vi "Pin Position Facade.vi"(0 "Data In":T6, 2 "Display State In":T3, 3 "Container State":T5) -> (6 "Data Out":T6, 7 "Display State Out":T3, 8 "Action":T2)   [LabVIEW 2013, in "Pin Position.xctl"]
uses:
  Pin Position.xctl
  Popups/Selected Pin Positions.ctl
  Pin Position Data.ctl
  lib/Data Access Objects/Metadata/Pin Positions.ctl
  <vilib>/_xctls/Container State.ctl
  Pin Position State.ctl
  lib/Data Access Objects/Application/Number Of LBCBs.ctl
  <vilib>/_xctls/Action.ctl
  lib/Data Access Objects/Metadata/Persistant DAO Actions.ctl
  lib/Data Access Objects/Metadata/LBCB Number.ctl
  <vilib>/_xctls/XControlSupport.lvlib
panel:
  in  "LBCB Position Tab":enum32{"LBCB 1", "LBCB 2"}(tab)
  in  "LBCB Position L1":T1
  in  "LBCB Position L2":T1
  # "Fixed"
  # "Platten"
  # "X"
  # "Z"
  # "X"
  # "Z"
  # "Y"
  # "Y"
  # "Fixed"
  # "Platten"
  # "X"
  # "Z"
  # "X"
  # "Z"
  # "Y"
  # "Y"
  # "Fixed"
  # "Platten"
  # "X"
  # "Z"
  # "X"
  # "Z"
  # "Y"
  # "Y"
  # "Fixed"
  # "Platten"
  # "X"
  # "Z"
  # "X"
  # "Z"
  # "Y"
  # "Y"
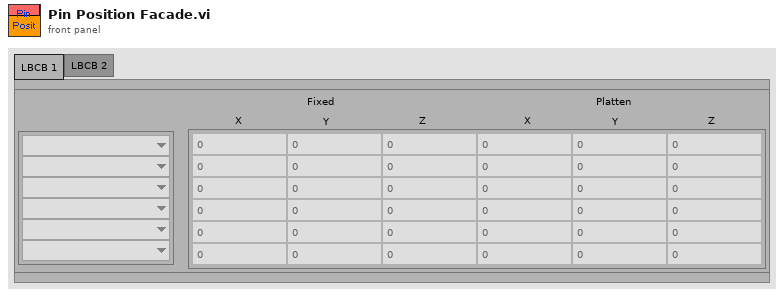
[diagram p1: front panel]
types:
  T1 = typedef "Selected Pin Positions.ctl" = cluster{"Pin Positions":dbl[][], "Row Labels":u16[]}
  T2 = typedef "XControlSupport.lvlib/Action.ctl" = cluster{"Data Changed?":bool, "State Changed?":bool, "Action Name":string}
  T3 = typedef "Pin Position.xctl/Pin Position State.ctl" = cluster{"Number of LBCBs":T4}
  T4 = typedef "Number Of LBCBs.ctl" = enum16{"1", "2"}
  T5 = typedef "XControlSupport.lvlib/Container State.ctl" = cluster{"Indicator?":bool, "Run Mode?":bool, " Refnum":refnum<vi>}
  T6 = typedef "Pin Position.xctl/Pin Position Data.ctl" = T7[]
  T7 = typedef "Pin Positions.ctl" = cluster{"Pin Positions":dbl[][], "Row Labels":string[]}
  T8 = enum8{"Enabled", "Disabled", "Disabled and Grayed Out"}
  T9 = typedef "LBCB Number.ctl" = enum16{"LBCB1", "LBCB2"}
  T10 = typedef "Persistant DAO Actions.ctl" = enum16{"Init", "Get", "Set", "Load", "Save"}
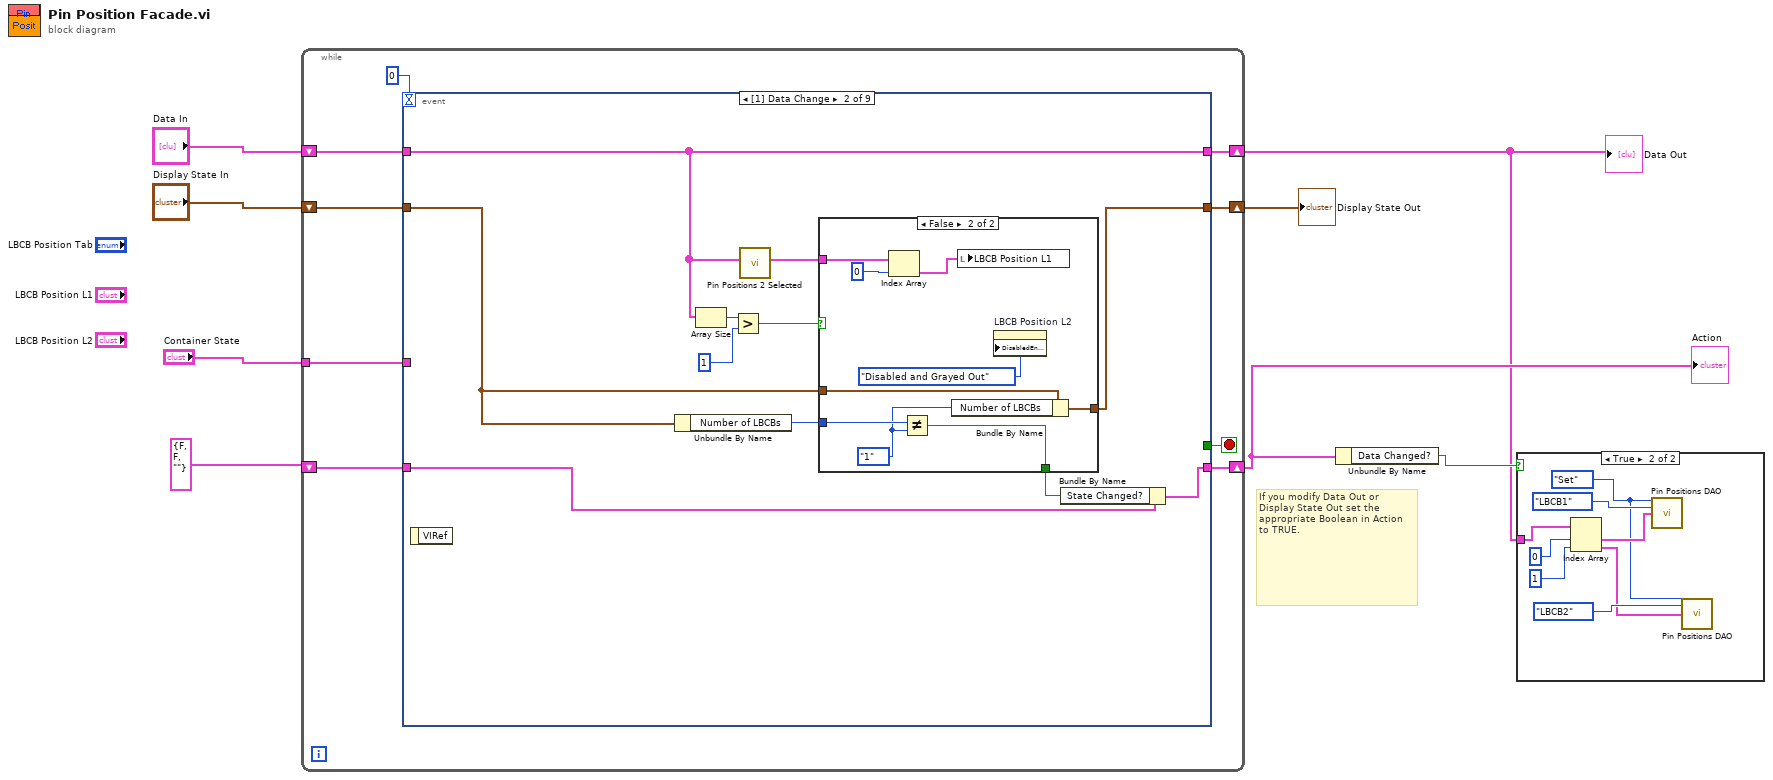
[diagram p0: block diagram]
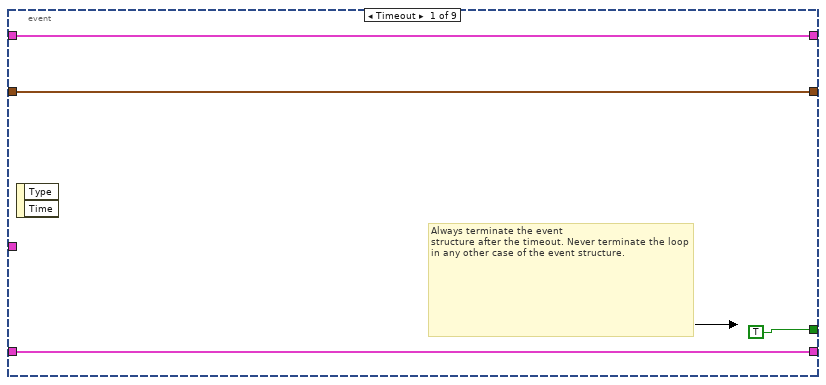
[diagram p3: hidden frame]
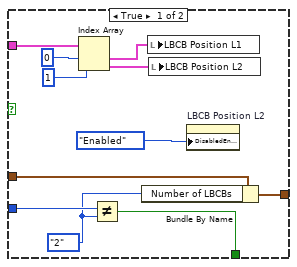
[diagram p4: hidden frame]
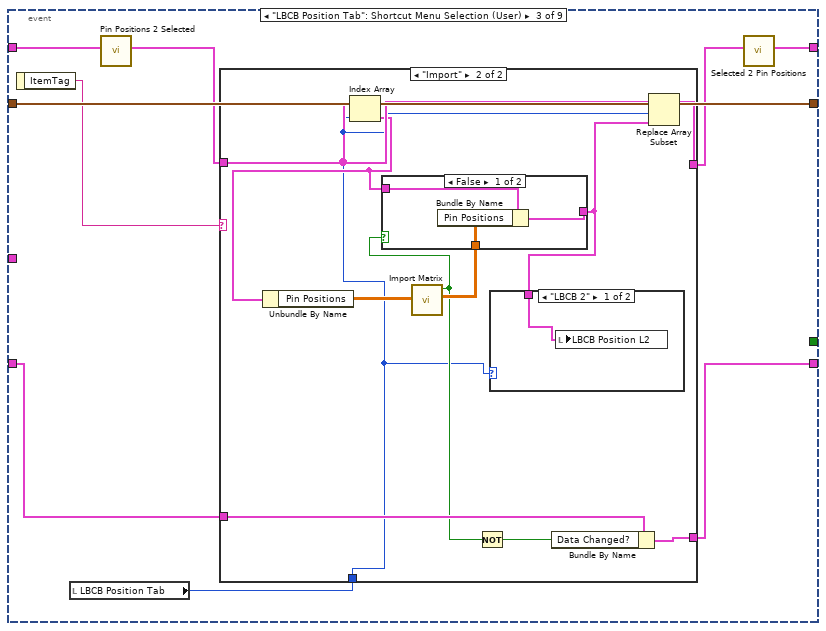
[diagram p5: hidden frame]
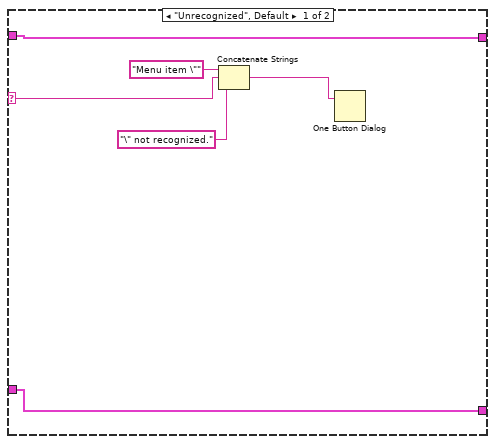
[diagram p6: hidden frame]
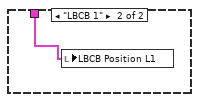
[diagram p7: hidden frame]
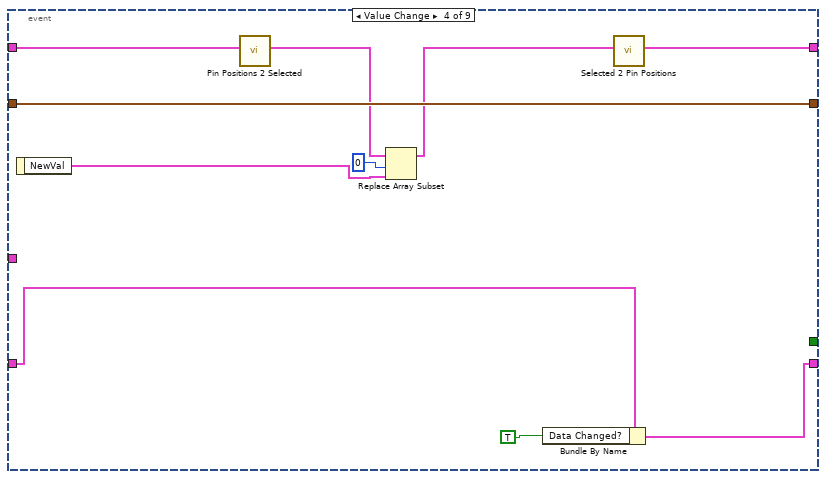
[diagram p9: hidden frame]
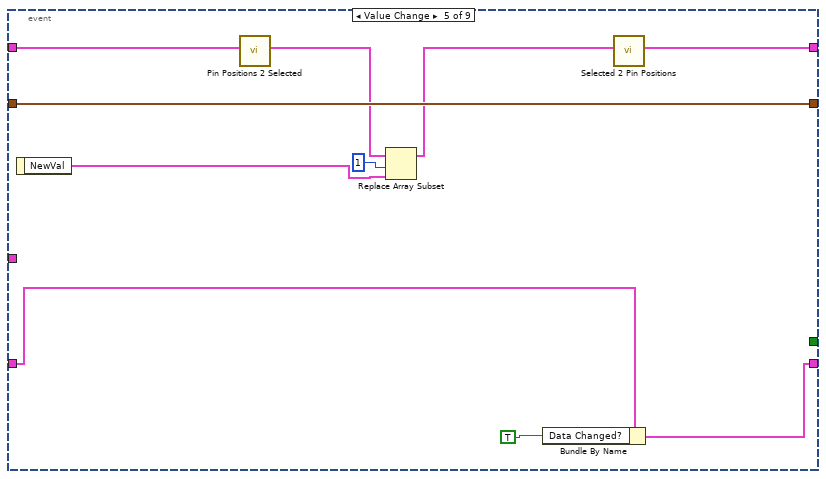
[diagram p10: hidden frame]
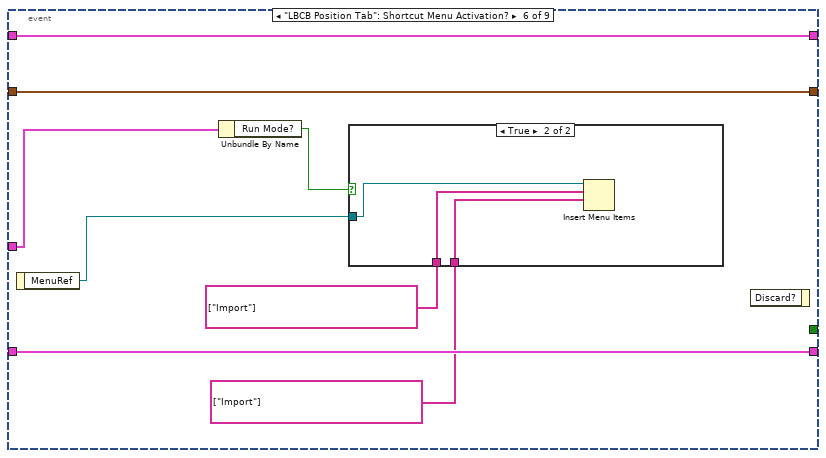
[diagram p11: hidden frame]
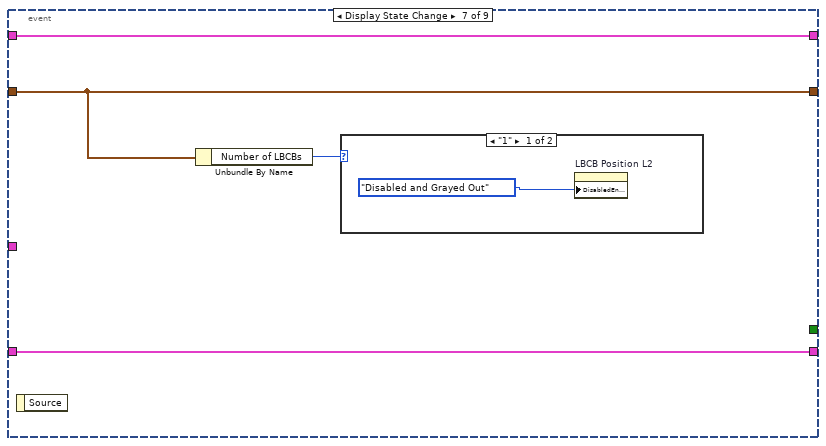
[diagram p13: hidden frame]
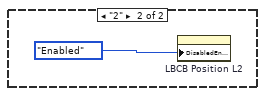
[diagram p14: hidden frame]
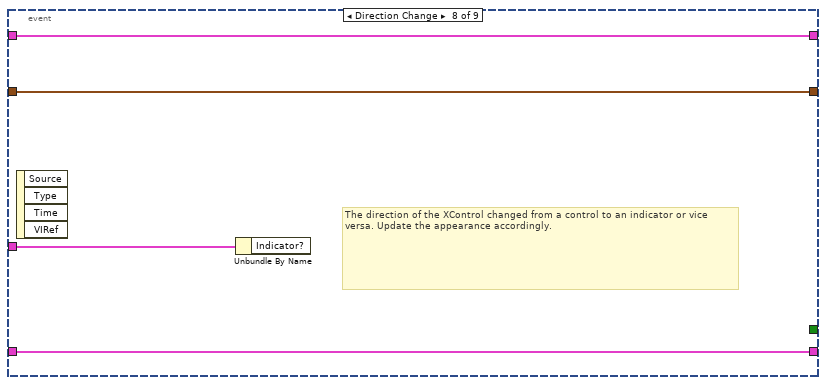
[diagram p15: hidden frame]
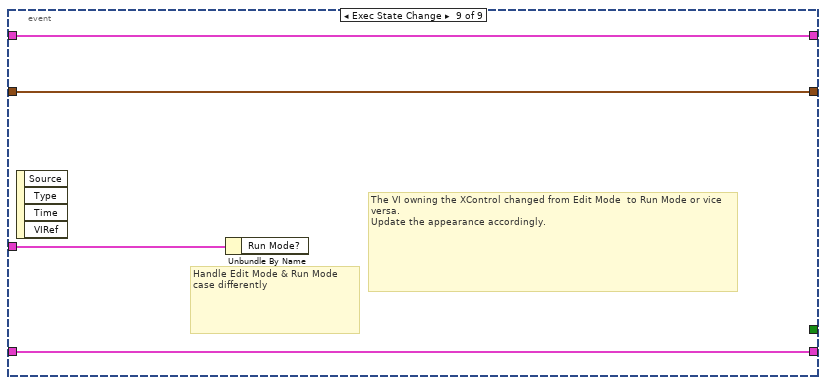
[diagram p16: hidden frame]
diagram:
  # "If you modify Data Out or\nDisplay State Out set the\nappropriate Boolean in Action\nto TRUE."
  n1 = while {
    shift-right: [w16] -> w6
    shift-left: "Display State In" -> [w17]
    tunnel: "Container State" -> [w13]
    shift-right: [w11] -> w1
    shift-left: "Data In" -> [w12]
    shift-right: [w9] -> w2
    shift-left: T2 {"Data Changed?"=FALSE, "State Changed?"=FALSE, "Action Name"=""} ("Action") -> [w10]
    stop <- w15 stop-if-true
    n2 = event shown="[1] Data Change" {
      selector: _ -> [_ _ _ _ _ _ _ _ _]
      dyn-events: _ -> [_ _ _ _ _ _ _ _ _]
      timeout: 0 -> [_ _ _ _ _ _ _ _ _]
      tunnel: w17 -> [w19 w24 w61 w94 w104 w112 w116 w124 w128]
      tunnel: [w19 w23 w61 w94 w104 w112 w116 w124 w128] -> w16
      tunnel: [TRUE _ _ _ _ _ _ _ _] -> w15
      tunnel: w13 -> [_ _ _ _ _ w106 _ w125 w129]
      tunnel: w12 -> [w18 w27 w58 w90 w100 w111 w119 w123 w127]
      tunnel: [w18 w27 w54 w87 w97 w111 w119 w123 w127] -> w11
      tunnel: [w20 w25 w56 w85 w95 w110 w118 w122 w126] -> w9
      tunnel: w10 -> [w20 w26 w60 w86 w96 w110 w118 w122 w126]
      event Timeout {
        # "Always terminate the event\nstructure after the timeout. Never terminate the loop in any other case of the event structure."
        n3 = event-data() -> ()  [unwired: 1 in, 2 out]
      }
      event Data Change {
        n4 = event-data() -> ()  [unwired: 1 in, 1 out]
        n5 = Unbundle By Name(w24) -> ("Number of LBCBs"=w31:T4)
        n6 = Array Size(array=w27) -> (size(s)=w28:i32)
        n7 = Greater?(x=w28, y=1) -> (0:w30:bool)
        n8 = call "Pin Positions 2 Selected.vi"("Pin"=w27) -> ("Selected"=w22:T1[])  [unwired: 10 in]
        n9 = case shown="False" w30 {
          tunnel: w22 -> [w43 w52]
          tunnel: w24 -> [w37 w48]
          tunnel: w31 -> [w38 w49]
          tunnel: [w35 w46] -> w32
          tunnel: [w34 w45] -> w23
          frame True {
            w36 = Number_Of_LBCBs."2" ("y")
            n10 = Index Array(array=w43, index #1=0 ("index"), index #2=1 ("index")) -> (element #1=w40:T1, element #2=w39:T1)
            n11 = Not Equal?(x=w38, y=w36) -> (x != y?=w35:bool)
            n12 = Bundle By Name(cluster=w37, "Number of LBCBs"=w36) -> (w34:T3)
            n13 = local write "LBCB Position L1"(w40) -> ()
            n14 = local write "LBCB Position L2"(w39) -> ()
            n15 = property on="LBCB Position L2" class="Clust (strict)"("DisabledEnum"=T8."Enabled" ("Disabled")) -> ()  [unwired: 2 in, 2 out]
          }
          frame False {
            w47 = Number_Of_LBCBs."1" ("y")
            n16 = Index Array(array=w52, index=0) -> (element=w50:T1)
            n17 = Not Equal?(x=w49, y=w47) -> (x != y?=w46:bool)
            n18 = Bundle By Name(cluster=w48, "Number of LBCBs"=w47) -> (w45:T3)
            n19 = local write "LBCB Position L1"(w50) -> ()
            n20 = property on="LBCB Position L2" class="Clust (strict)"("DisabledEnum"=T8."Disabled and Grayed Out" ("Disabled")) -> ()  [unwired: 2 in, 2 out]
          }
        }
        n21 = Bundle By Name(cluster=w26, "State Changed?"=w32) -> (w25:T2)
      }
      event "LBCB Position Tab": Shortcut Menu Selection (User) {
        n22 = event-data() -> ("ItemTag"=w59:string)  [unwired: 1 in]
        n23 = local read "LBCB Position Tab"() -> (w53:enum32{"LBCB 1", "LBCB 2"})
        n24 = call "Pin Positions 2 Selected.vi"("Pin"=w58) -> ("Selected"=w55:T1[])  [unwired: 10 in]
        n25 = case shown="\"Import\"" w59 {
          selector: w59 -> [w65 _]
          tunnel: w55 -> [w63 w78]
          tunnel: [w63 w77] -> w57
          tunnel: w60 -> [w62 w73]
          tunnel: [w62 w72] -> w56
          tunnel: w53 -> [_ w68]
          frame "Unrecognized", Default {
            n26 = Concatenate Strings("Menu item \"" ("string"), w65, "\" not recognized." ("string")) -> (w64:string)
            n27 = One Button Dialog(message=w64) -> ()  [unwired: 1 in, 1 out]
          }
          frame "Import" {
            n28 = Index Array(array=w78, index=w68) -> (element=w76:T1)
            n29 = Unbundle By Name(w76) -> ("Pin Positions"=w75:dbl[][])
            n30 = call "Import Matrix.vi"("PinPositions In"=w75) -> ("PinPositions Out"=w74:dbl[][], "Canceled"=w71:bool)  [unwired: 9 in]
            n31 = case shown="False" w71 {
              tunnel: [w83 w84] -> w69
              tunnel: w76 -> [w82 w84]
              tunnel: w74 -> [w81 _]
              frame False {
                n32 = Bundle By Name(cluster=w82, "Pin Positions"=w81) -> (w83:T1)
              }
              frame True {
              }
            }
            n33 = Not(x=w71) -> (.not. x?=w70:bool)
            n34 = case shown="\"LBCB 2\"" w68 {
              tunnel: w69 -> [w79 w80]
              frame "LBCB 2" {
                n35 = local write "LBCB Position L2"(w79) -> ()
              }
              frame "LBCB 1" {
                n36 = local write "LBCB Position L1"(w80) -> ()
              }
            }
            n37 = Bundle By Name(cluster=w73, "Data Changed?"=w70) -> (w72:T2)
            n38 = Replace Array Subset(array=w78, new element=w69, index=w68) -> (w77:T1[])
          }
        }
        n39 = call "Selected 2 Pin Positions.vi"("Selected"=w57) -> ("Pin"=w54:T7[])  [unwired: 10 in]
      }
      event Value Change {
        n40 = event-data() -> ("NewVal"=w91:T1)  [unwired: 1 in]
        n41 = call "Pin Positions 2 Selected.vi"("Pin"=w90) -> ("Selected"=w89:T1[])  [unwired: 10 in]
        n42 = Replace Array Subset(array=w89, new element=w91, index=0) -> (w88:T1[])
        n43 = Bundle By Name(cluster=w86, "Data Changed?"=TRUE) -> (w85:T2)
        n44 = call "Selected 2 Pin Positions.vi"("Selected"=w88) -> ("Pin"=w87:T7[])  [unwired: 10 in]
      }
      event Value Change {
        n45 = event-data() -> ("NewVal"=w101:T1)  [unwired: 1 in]
        n46 = call "Pin Positions 2 Selected.vi"("Pin"=w100) -> ("Selected"=w99:T1[])  [unwired: 10 in]
        n47 = Replace Array Subset(array=w99, new element=w101, index=1) -> (w98:T1[])
        n48 = Bundle By Name(cluster=w96, "Data Changed?"=TRUE) -> (w95:T2)
        n49 = call "Selected 2 Pin Positions.vi"("Selected"=w98) -> ("Pin"=w97:T7[])  [unwired: 10 in]
      }
      event "LBCB Position Tab": Shortcut Menu Activation? {
        n50 = event-data() -> ("MenuRef"=w105:refnum<k9>)  [unwired: 1 in]
        n51 = Unbundle By Name(w106) -> ("Run Mode?"=w107:bool)
        n52 = case shown="True" w107 {
          tunnel: w105 -> [_ w115]
          tunnel: string[] ["Import"] -> [_ w114]
          tunnel: string[] ["Import"] -> [_ w113]
          frame False {
          }
          frame True {
            n53 = Insert Menu Items(7:w113, 8:w114, 9:w115) -> ()  [unwired: 3 in, 3 out]
          }
        }
        n54 = event-data() -> ()  [unwired: 2 in, 1 out]
      }
      event Display State Change {
        n55 = event-data() -> ()  [unwired: 1 in, 1 out]
        n56 = Unbundle By Name(w116) -> ("Number of LBCBs"=w117:T4)
        n57 = case shown="\"1\"" w117 {
          frame "1" {
            n58 = property on="LBCB Position L2" class="Clust (strict)"("DisabledEnum"=T8."Disabled and Grayed Out" ("Disabled")) -> ()  [unwired: 2 in, 2 out]
          }
          frame "2" {
            n59 = property on="LBCB Position L2" class="Clust (strict)"("DisabledEnum"=T8."Enabled" ("Disabled")) -> ()  [unwired: 2 in, 2 out]
          }
        }
      }
      event Direction Change {
        # "The direction of the XControl changed from a control to an indicator or vice versa. Update the appearance accordingly."
        n60 = event-data() -> ()  [unwired: 1 in, 4 out]
        n61 = Unbundle By Name(w125) -> ()  [unwired: 1 out]
      }
      event Exec State Change {
        # "The VI owning the XControl changed from Edit Mode  to Run Mode or vice versa.\nUpdate the appearance accordingly."
        # "Handle Edit Mode & Run Mode\ncase differently"
        n62 = event-data() -> ()  [unwired: 1 in, 4 out]
        n63 = Unbundle By Name(w129) -> ()  [unwired: 1 out]
      }
    }
  }
  "Display State Out" <- w6
  "Data Out" <- w1
  "Action" <- w2
  n64 = Unbundle By Name(w2) -> ("Data Changed?"=w3:bool)
  n65 = case shown="True" w3 {
    tunnel: w1 -> [_ w134]
    frame False {
    }
    frame True {
      w132 = Persistant_DAO_Actions."Set" ("LBCB Settings Actions")
      n66 = Index Array(array=w134, index #1=0 ("index"), index #2=1 ("index")) -> (element #1=w133:T7, element #2=w130:T7)
      n67 = call "Pin Positions DAO.vi"("LBCB Settings Actions"=w132, "LBCB Number"=LBCB_Number."LBCB1", "LBCB Pins In"=w133) -> ()  [unwired: 10 in, 3 out]
      n68 = call "Pin Positions DAO.vi"("LBCB Settings Actions"=w132, "LBCB Number"=LBCB_Number."LBCB2", "LBCB Pins In"=w130) -> ()  [unwired: 10 in, 3 out]
    }
  }
